vi "Catch Nested Value Update.vi"(8 "error in (no error)":errorcluster, 10 "Nested Value Update Msg":refnum<class "Nested Value Update Msg.lvclass">, 11 "IViewable In":refnum<class "IViewable.lvclass">) -> (0 "error out":errorcluster, 3 "IViewable Out":refnum<class "IViewable.lvclass">)   [LabVIEW 2020, in "MVA Framework.lvlib" / "IViewable.lvlib" / "IViewable.lvclass"]
doc: "捕获嵌套值更新"
uses:
  IViewable.lvclass
  C:/Program Files/National Instruments/LabVIEW 2020/vi.lib/ActorFramework/Actor/Actor.lvclass
  IViewable Messages/Catch Nested Value Change Msg/Nested Value Update Msg.lvclass
  C:/Program Files/National Instruments/LabVIEW 2020/vi.lib/ActorFramework/Message/Message.lvclass
  <vilib>/ActorFramework/Actor/Actor.lvclass/Actor.ctl
  <vilib>/ActorFramework/Message Enqueuer/Message Enqueuer.lvclass/Message Enqueuer.ctl
  <vilib>/ActorFramework/Message Priority Queue/Priority Enqueue.vi
  <vilib>/ActorFramework/Actor/Actor.lvclass
  <vilib>/ActorFramework/Message Enqueuer/Message Enqueuer.lvclass
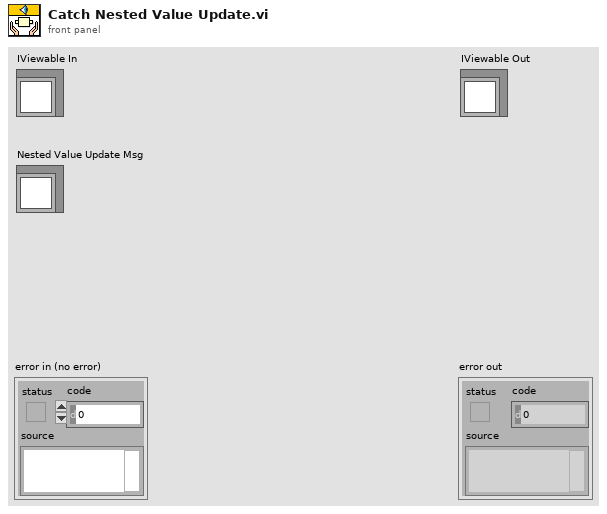
[diagram p1: front panel]
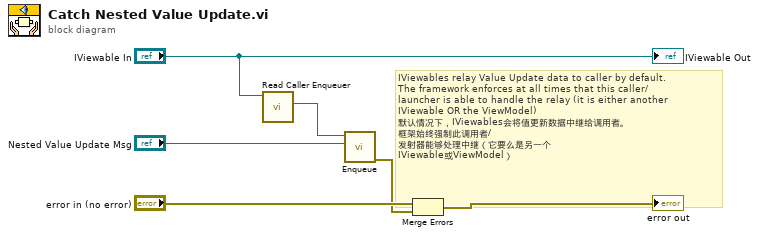
[diagram p0: block diagram]
diagram:
  # "IViewables relay Value Update data to caller by default.\nThe framework enforces at all times that this caller/\nlauncher is able to handle the relay (it is either another\nIViewable OR the ViewModel)\n默认情况下，IViewables会将值更新数据中继给调用者。\n框架始终强制此调用者/\n发射器能够处理中继（它要么是另一个\nIViewable或ViewModel）"
  n1 = call <vilib>:"Read Caller Enqueuer.vi"("Actor"="IViewable In") -> ("Caller Enqueuer"=w3:refnum<class "Message Enqueuer.lvclass">)  [unwired: 10 in]
  n2 = call <vilib>:"Enqueue.vi"("Message"="Nested Value Update Msg", "Message Enqueuer in"=w3) -> ("error out"=w1:errorcluster)  [unwired: 8 in, 1 out]
  n3 = Merge Errors("error in (no error)", w1) -> (→"error out":errorcluster)
  "IViewable Out" <- "IViewable In"
